vi "Write Value.vi"(8 "error in (no error)":errorcluster, 10 "Value":dbl[](array[numeric]), 11 "Double Parameter in":refnum<class "Double Array Parameter.lvclass">) -> (0 "error out":errorcluster, 3 "Double Parameter out":refnum<class "Double Array Parameter.lvclass">)   [LabVIEW 2019, in "CD Parameter Manager API.lvlib" / "Double Array Parameter.lvclass"]
uses:
  Double Array Parameter.lvclass
  Double Array Parameter.lvclass/Double Array Parameter.ctl
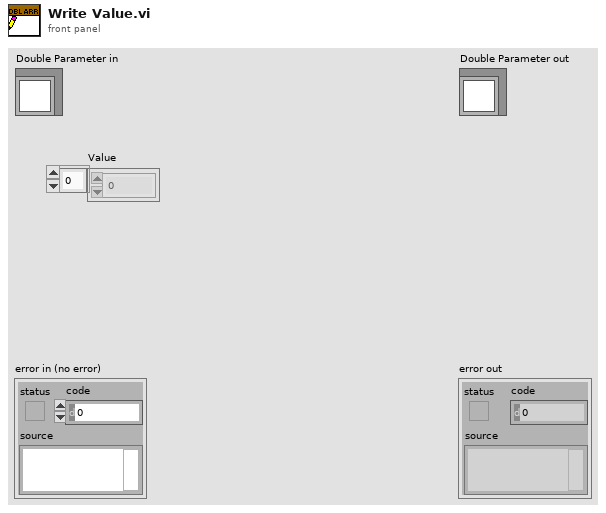
[diagram p1: front panel]
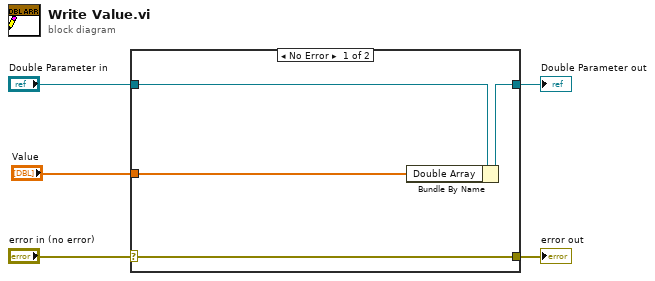
[diagram p0: block diagram]
diagram:
  n1 = case shown="No Error" "error in (no error)" {
    selector: "error in (no error)" -> [w9 w10]
    tunnel: [w9 w10] -> w4
    tunnel: [w7 w11] -> w2
    tunnel: "Double Parameter in" -> [w8 w11]
    tunnel: "Value" -> [w6 _]
    frame No Error {
      n2 = Bundle By Name(cluster=w8, "Double Array"=w6) -> (w7:refnum<class "Double Array Parameter.lvclass">)
    }
    frame Error {
    }
  }
  "error out" <- w4
  "Double Parameter out" <- w2
